vi "Resolve File.vi"(8 "error in (no error)":errorcluster, 10 "File in":T1, 11 "CubeLogger in":refnum<class "CubeLogger.lvclass">) -> (0 "error out":errorcluster, 2 "File out":T1, 3 "CubeLogger out":refnum<class "CubeLogger.lvclass">)   [LabVIEW 2018]
uses:
  CubeLogger.lvclass
  File.ctl
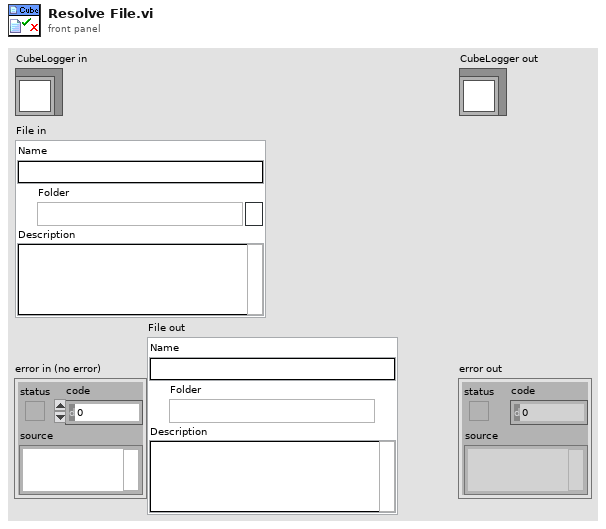
[diagram p1: front panel]
types:
  T1 = typedef "CubeLogger.lvclass/File.ctl" = cluster{"Name":string, "Folder":path, "Description":string}
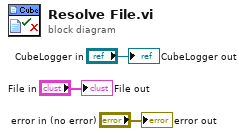
[diagram p0: block diagram]
diagram:
  "error out" <- "error in (no error)"
  "CubeLogger out" <- "CubeLogger in"
  "File out" <- "File in"
